vi "8.vi"() -> ()   [LabVIEW 2017, in "ErrorStructureDrawer-Tests.lvlib"]
uses:
  ErrorStructureDrawer-Tests.lvlib
panel:
  out "path":path
  out "error out":errorcluster
  in  "error in":errorcluster
  in  "file path (use dialog)":path
  in  "operation (0:open)":T1(ring)
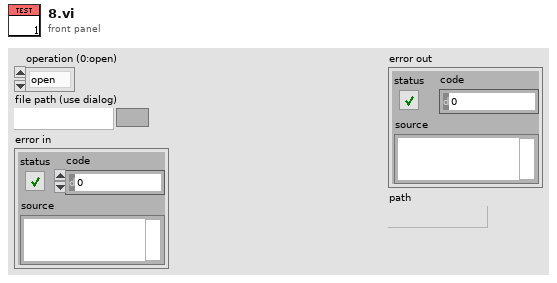
[diagram p1: front panel]
types:
  T1 = enum16{"open", "replace", "create", "open or create", "replace or create", "replace or create with confirmation"}
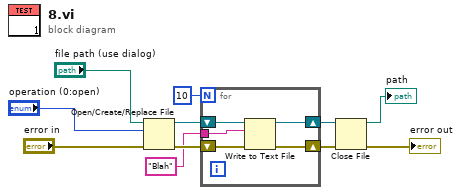
[diagram p0: block diagram]
diagram:
  n1 = Open/Create/Replace File(file path (use dialog)="file path (use dialog)", error in="error in", operation (0:open)="operation (0:open)") -> (refnum out=w11:refnum<file>, error out=w9:errorcluster)  [unwired: 3 in, 1 out]
  n2 = for {
    N: 10 -> [_]
    shift-right: [w15] -> w10
    shift-left: w11 -> [w16]
    shift-right: [w13] -> w8
    shift-left: w9 -> [w14]
    tunnel: "Blah" -> [w12]
    n3 = Write to Text File(file (use dialog)=w16, text=w12, error in=w14) -> (refnum out=w15:refnum<file>, error out=w13:errorcluster)  [unwired: 1 in, 1 out]
  }
  n4 = Close File(refnum=w10, error in=w8) -> (path=→"path":path, error out=→"error out":errorcluster)
